vi "test Major Frame Instructions.vi"(8 "error in (no error)":errorcluster, 11 "BC Major Frame in":refnum<class "BC Major Frame.lvclass">) -> (0 "error out":errorcluster, 3 "BC Major Frame out":refnum<class "BC Major Frame.lvclass">)   [LabVIEW 2016, in "BC Major Frame.lvclass"]
uses:
  BC Major Frame.lvclass
  Data Pointers.ctl
  BC Major Frame.lvclass/BC Major Frame.ctl
  Dependencies/Registry/Registry.lvclass/Registry.ctl
  Frames & Messages/TypeDefs/BC Op Codes - Verbose.ctl
  Frames & Messages/TypeDefs/BC Condition Codes.ctl
  PPLs/FPGA Interface.lvlibp/FPGA Interface/FPGA Interface.lvclass
  BCI-1553 API.lvlib
  Dependencies/Registry/Registry.lvclass
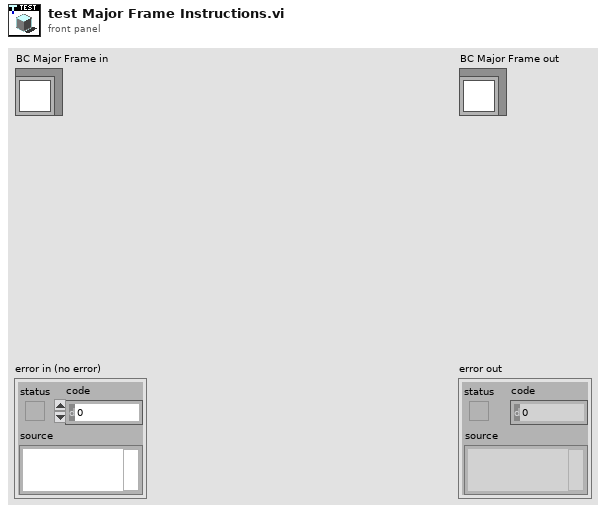
[diagram p1: front panel]
types:
  T1 = typedef "Data Pointers.ctl" = cluster{"Major Command Pointer":u16, "Major Data Pointer":u16, "Minor Command Pointer":u16, "Minor Data Pointer":u16}
  T2 = typedef "BCI-1553 API.lvlib/BC Condition Codes.ctl" = enum16{"GP0 == 1 || LT", "GP1 == 1 || NE", "GP2 == 1", "GP3 == 1", "GP4 == 1", "GP5 == 1", "GP6 == 1", "GP7 == 1", "NORESP", "FMTERR", "GOODBLOCK", "MSKSTATSET", "BADMSG", "1RETRY", "2RETRY", "ALWAYS"}
  T3 = typedef "BCI-1553 API.lvlib/BC Op Codes - Verbose.ctl" = enum16{"EXECUTE MSG", "EXECUTE MSG GO", "JUMP", "CALL SUBROUTINE", "RETURN", "INTERRUPT REQUEST", "HALT", "DELAY", "WAIT FRAME TIMER = 0", "COMPARE FRAME TIMER", "COMPARE MSG TIMER", "LOAD TIME TAG CTR", "LOAD TIME TAG CTR HI", "LOAD FRAME TIMER", "START FRAME TIMER", "PUSH TIME TAG COUNT", "PUSH TIME TAG COUNT HI", "PUSH TIME TAG COUNT BOTH", "PUSH BLOCK STATUS WORD", "PUSH CURRENT VALUE", "PUSH INDIRECT", "WAIT EXT TRIGGER", "EXECUTE AND FLIP", "EXECUTE, FLIP, GO", "WRITE VALUE TO WMI", "WRITE VALUE TO MEM", "DECREMENT RAM, SKIP", "FLAG"}
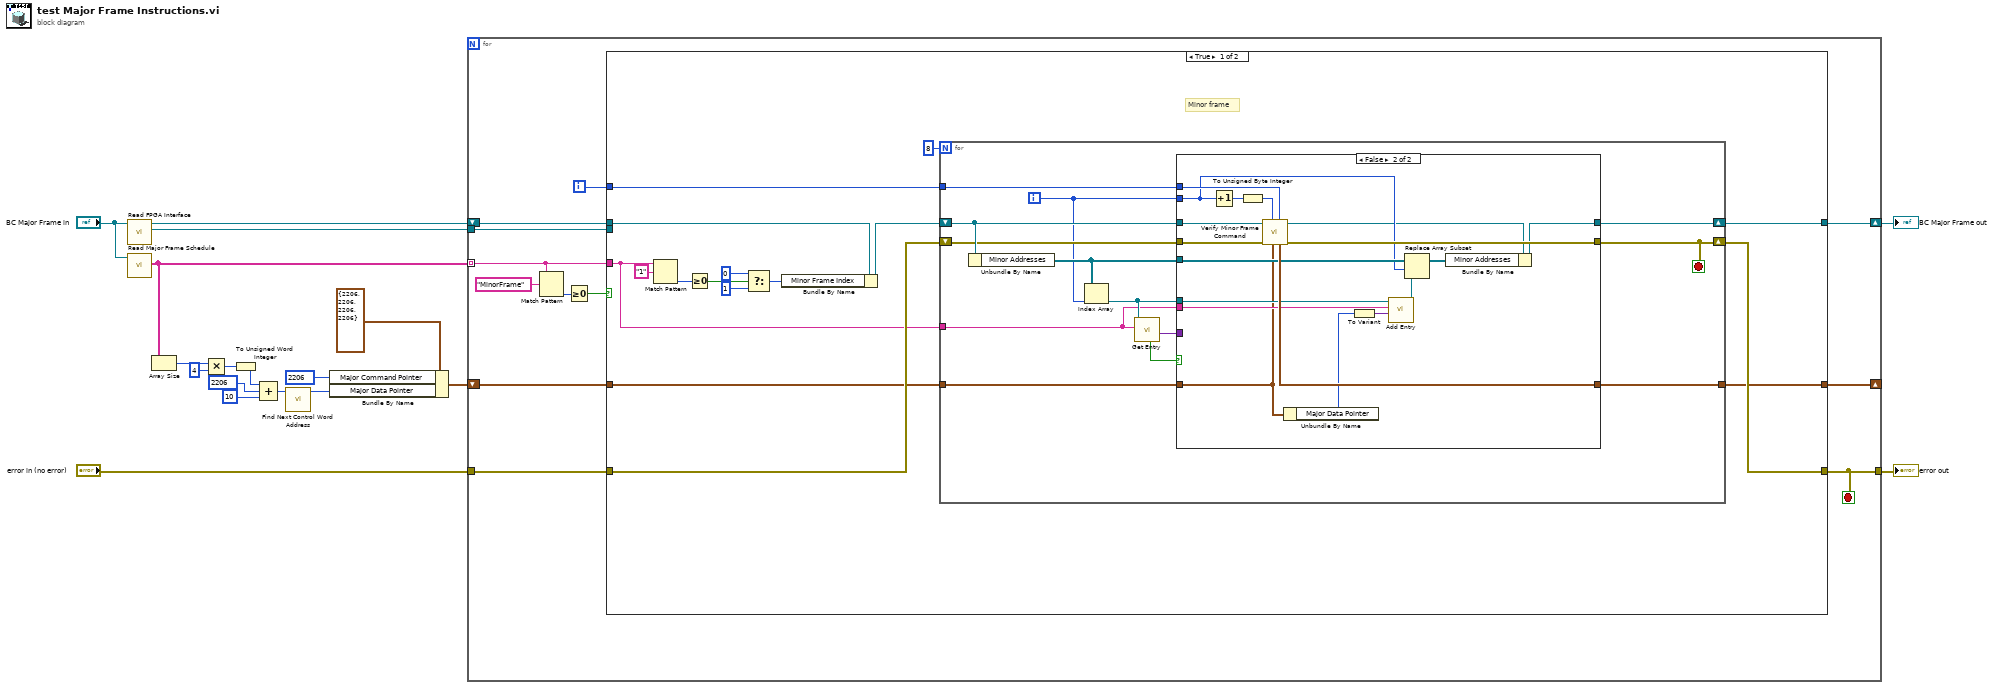
[diagram p0: block diagram]
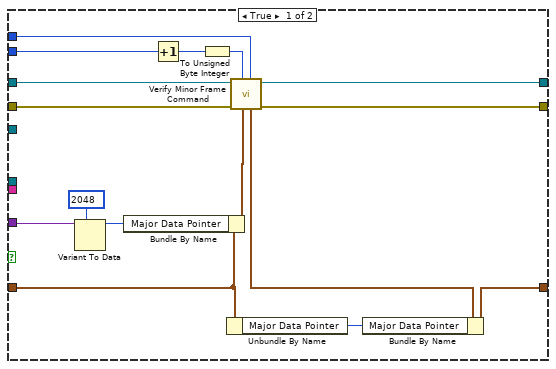
[diagram p2: hidden frame]
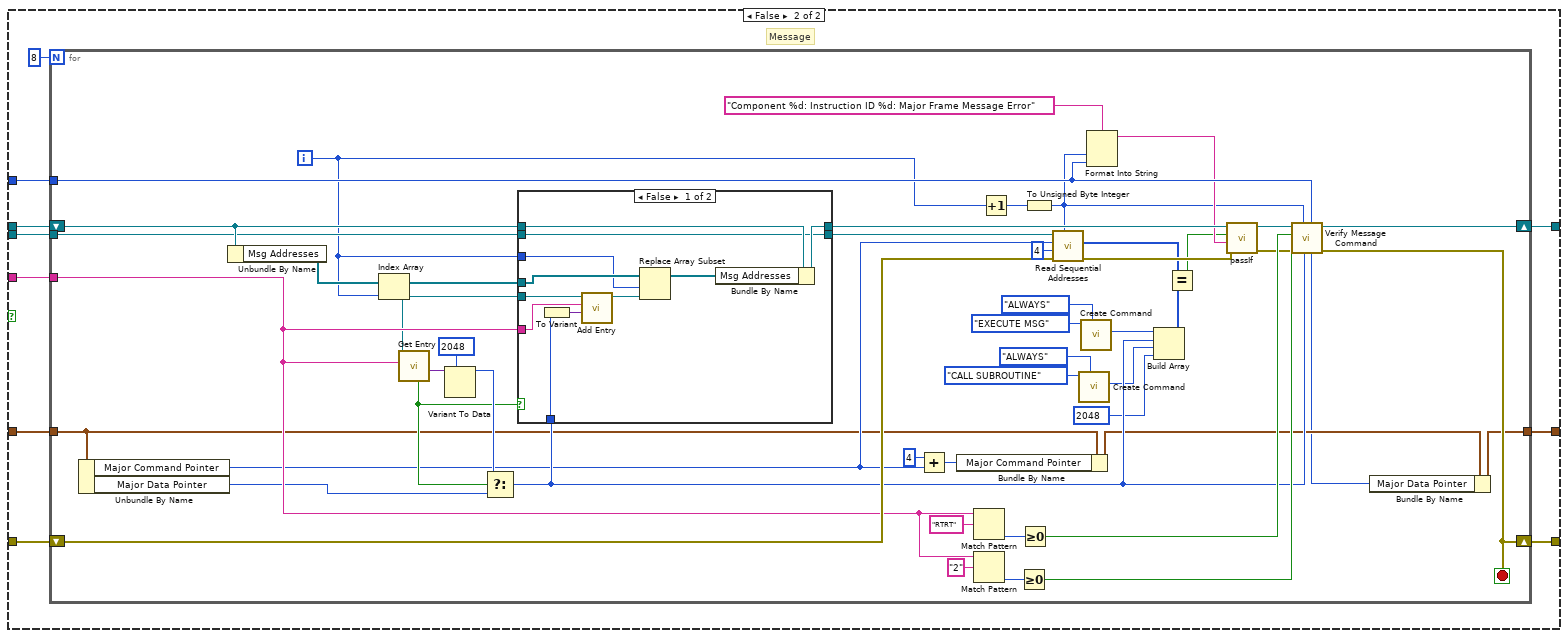
[diagram p3: hidden frame]
diagram:
  n1 = call-dynamic "Read FPGA Interface.vi"("1553 Test in"="BC Major Frame in") -> ("FPGA Interface"=w14:refnum<class "FPGA Interface.lvclass">, "1553 Test out"=w15:refnum<class "BC Major Frame.lvclass">)  [unwired: 8 in, 1 out]
  n2 = call-dynamic "Read Major Frame Schedule.vi"("1553 Test in"="BC Major Frame in") -> ("Major Frame Schedule"=w12:string[])  [unwired: 8 in, 2 out]
  n3 = Array Size(array=w12) -> (size(s)=w10:i32)
  n4 = Multiply(x=w10, y=4) -> (x*y=w8:i32)
  n5 = To Unsigned Word Integer(number=w8) -> (unsigned 16bit integer=w7:u16)
  n6 = Compound Arithmetic op=ADD(w7, u16 2206, u16 10 ("y")) -> (w5:u16)
  n7 = call "Find Next Control Word Address.vi"("Starting Address"=w5) -> ("0xHHHX Address"=w2:u16)  [unwired: 10 in]
  n8 = Bundle By Name(cluster=T1 {"Major Command Pointer"=2206, "Major Data Pointer"=2206, "Minor Command Pointer"=2206, "Minor Data Pointer"=2206}, "Major Command Pointer"=u16 2206, "Major Data Pointer"=w2) -> (w1:T1)
  n9 = for {
    shift-right: [w29] -> w18
    shift-left: w15 -> [w30]
    tunnel: "error in (no error)" -> [w28]
    tunnel: [w26] -> w16
    tunnel: w14 -> [w27]
    tunnel: w12 -> [w22] mode=indexing
    shift-right: [w19] -> _
    shift-left: w1 -> [w20]
    i -> [w21]
    stop <- w26 stop-if-true
    n10 = Match Pattern(string=w22, regular expression="MinorFrame") -> (offset past match=w24:i32)  [unwired: 1 in, 3 out]
    n11 = Greater Or Equal To 0?(x=w24) -> (x >= 0?=w23:bool)
    n12 = case shown="True" w23 {
      tunnel: w30 -> [w42 w99]
      tunnel: [w46 w103] -> w29
      tunnel: w28 -> [w44 w101]
      tunnel: [w43 w100] -> w26
      tunnel: w27 -> [_ w98]
      tunnel: w22 -> [w31 w97]
      tunnel: w21 -> [w45 w102]
      tunnel: w20 -> [w33 w95]
      tunnel: [w32 w94] -> w19
      frame True {
        # "Minor frame"
        n13 = Match Pattern(string=w31, regular expression="1") -> (offset past match=w39:i32)  [unwired: 1 in, 3 out]
        n14 = Greater Or Equal To 0?(x=w39) -> (x >= 0?=w38:bool)
        n15 = Select(t=0 ("Minor Frame Index"), s=w38, f=1 ("Minor Frame Index")) -> (s? t:f=w36:i32)
        n16 = Bundle By Name(cluster=w42, "Minor Frame Index"=w36) -> (w41:refnum<class "BC Major Frame.lvclass">)
        n17 = for {
          N: 8 -> [_]
          tunnel: w45 -> [w56]
          shift-right: [w58] -> w43
          shift-left: w44 -> [w53]
          shift-right: [w59] -> w46
          shift-left: w41 -> [w54]
          tunnel: w33 -> [w55]
          tunnel: [w57] -> w32
          tunnel: w31 -> [w47]
          i -> [w48]
          stop <- w58 stop-if-true
          n18 = Unbundle By Name(w54) -> ("Minor Addresses"=w49:refnum<class "Registry.lvclass">[])
          n19 = Index Array(array=w49, index=w48) -> (element=w50:refnum<class "Registry.lvclass">)
          n20 = call "Get Entry.vi"("Key"=w47, "Registry in"=w50) -> ("Value"=w51:variant, "Found?"=w52:bool)  [unwired: 6 in, 2 out]
          n21 = case shown="False" w52 {
            tunnel: [w75 w82] -> w59
            tunnel: [w72 w91] -> w58
            tunnel: [w61 w88] -> w57
            tunnel: w56 -> [w71 w86]
            tunnel: w55 -> [w63 w76]
            tunnel: w54 -> [w66 w89]
            tunnel: w53 -> [w70 w90]
            tunnel: w51 -> [w68 _]
            tunnel: w50 -> [_ w80]
            tunnel: w48 -> [w67 w85]
            tunnel: w49 -> [_ w87]
            tunnel: w47 -> [_ w78]
            frame True {
              n22 = Variant To Data(type=u16 2048, Variant=w68) -> (data=w65:u16)  [unwired: 1 in, 1 out]
              n23 = Bundle By Name(cluster=w63, "Major Data Pointer"=w65) -> (w64:T1)
              n24 = Increment(x=w67) -> (x+1=w73:i32)
              n25 = To Unsigned Byte Integer(number=w73) -> (unsigned 8bit integer=w74:u8)
              n26 = Unbundle By Name(w63) -> ("Major Data Pointer"=w60:u16)
              n27 = call "Verify Minor Frame Command.vi"("Instruction ID"=w71, "Pointers"=w64, "Target IC (1-8)"=w74, "error in (no error)"=w70, "BC Major Frame in"=w66) -> ("error out"=w72:errorcluster, "BC Major Frame out"=w75:refnum<class "BC Major Frame.lvclass">, "Pointers out"=w62:T1)  [unwired: 4 in]
              n28 = Bundle By Name(cluster=w62, "Major Data Pointer"=w60) -> (w61:T1)
            }
            frame False {
              n29 = Increment(x=w85) -> (x+1=w92:i32)
              n30 = To Unsigned Byte Integer(number=w92) -> (unsigned 8bit integer=w93:u8)
              n31 = call "Verify Minor Frame Command.vi"("Instruction ID"=w86, "Pointers"=w76, "Target IC (1-8)"=w93, "error in (no error)"=w90, "BC Major Frame in"=w89) -> ("error out"=w91:errorcluster, "BC Major Frame out"=w83:refnum<class "BC Major Frame.lvclass">, "Pointers out"=w88:T1)  [unwired: 4 in]
              n32 = Unbundle By Name(w76) -> ("Major Data Pointer"=w79:u16)
              n33 = To Variant(anything=w79) -> (Variant=w81:variant)
              n34 = call "Add Entry.vi"("Value"=w81, "Key"=w78, "Registry in"=w80) -> ("Registry out"=w77:refnum<class "Registry.lvclass">)  [unwired: 6 in, 2 out]
              n35 = Replace Array Subset(array=w87, new element=w77, index=w85) -> (w84:refnum<class "Registry.lvclass">[])
              n36 = Bundle By Name(cluster=w83, "Minor Addresses"=w84) -> (w82:refnum<class "BC Major Frame.lvclass">)
            }
          }
        }
      }
      frame False {
        # "Message"
        n37 = for {
          N: 8 -> [_]
          tunnel: w102 -> [w151]
          tunnel: w98 -> [w137]
          tunnel: w97 -> [w134]
          shift-right: [w111] -> w100
          shift-left: w101 -> [w150]
          shift-right: [w152] -> w103
          shift-left: w99 -> [w138]
          tunnel: w95 -> [w107]
          tunnel: [w105] -> w94
          i -> [w112]
          stop <- w111 stop-if-true
          n38 = Unbundle By Name(w107) -> ("Major Command Pointer"=w109:u16, "Major Data Pointer"=w110:u16)
          n39 = Unbundle By Name(w138) -> ("Msg Addresses"=w114:refnum<class "Registry.lvclass">[])
          n40 = Index Array(array=w114, index=w112) -> (element=w113:refnum<class "Registry.lvclass">)
          n41 = call "Get Entry.vi"("Key"=w134, "Registry in"=w113) -> ("Value"=w142:variant, "Found?"=w139:bool)  [unwired: 6 in, 2 out]
          n42 = Variant To Data(type=u16 2048, Variant=w142) -> (data=w140:u16)  [unwired: 1 in, 1 out]
          n43 = Select(t=w140, s=w139, f=w110) -> (s? t:f=w133:u16)
          n44 = case shown="False" w139 {
            tunnel: w114 -> [w155 _]
            tunnel: w134 -> [w163 _]
            tunnel: w133 -> [w162 _]
            tunnel: [w158 w165] -> w136
            tunnel: w137 -> [w158 w165]
            tunnel: [w159 w164] -> w135
            tunnel: w138 -> [w160 w164]
            tunnel: w113 -> [w157 _]
            tunnel: w112 -> [w153 _]
            frame False {
              n45 = To Variant(anything=w162) -> (Variant=w161:variant)
              n46 = call "Add Entry.vi"("Value"=w161, "Key"=w163, "Registry in"=w157) -> ("Registry out"=w156:refnum<class "Registry.lvclass">)  [unwired: 6 in, 2 out]
              n47 = Replace Array Subset(array=w155, new element=w156, index=w153) -> (w154:refnum<class "Registry.lvclass">[])
              n48 = Bundle By Name(cluster=w160, "Msg Addresses"=w154) -> (w159:refnum<class "BC Major Frame.lvclass">)
            }
            frame True {
            }
          }
          n49 = Add(x=u16 4 ("y"), y=w109) -> (x+y=w108:u16)
          n50 = Bundle By Name(cluster=w107, "Major Command Pointer"=w108) -> (w106:T1)
          n51 = Match Pattern(string=w134, regular expression="RTRT") -> (offset past match=w145:i32)  [unwired: 1 in, 3 out]
          n52 = Match Pattern(string=w134, regular expression="2") -> (offset past match=w148:i32)  [unwired: 1 in, 3 out]
          n53 = Increment(x=w112) -> (x+1=w115:i32)
          n54 = Greater Or Equal To 0?(x=w148) -> (x >= 0?=w143:bool)
          n55 = Greater Or Equal To 0?(x=w145) -> (x >= 0?=w144:bool)
          n56 = To Unsigned Byte Integer(number=w115) -> (unsigned 8bit integer=w127:u8)
          n57 = call-dynamic "Read Sequential Addresses.vi"("Target IC (1-8)"=w127, "error in (no error)"=w150, "Addresses to Read"=u16 4, "Starting Address"=w109, "FPGA Interface in"=w136) -> ("error out"=w128:errorcluster, "Data"=w118:u16[])  [unwired: 5 in]
          n58 = call "Create Command.vi"("Condition"=BC_Condition_Codes."ALWAYS", "Op Code"=BC_Op_Codes_-_Verbose."CALL SUBROUTINE") -> ("Instruction"=w121:u16)  [unwired: 8 in, 1 out]
          n59 = call "Create Command.vi"("Condition"=BC_Condition_Codes."ALWAYS", "Op Code"=BC_Op_Codes_-_Verbose."EXECUTE MSG") -> ("Instruction"=w120:u16)  [unwired: 8 in, 1 out]
          n60 = Format Into String(format string="Component %d: Instruction ID %d: Major Frame Message Error" ("message (\"\")"), w127, w151) -> (resulting string=w129:string)  [unwired: 2 in, 1 out]
          n61 = Build Array(w120, w133, w121, u16 2048) -> (w119:u16[])
          n62 = Equal?(x=w118, y=w119) -> (x = y?=w116:bool)
          n63 = call-dynamic "passIf.vi"("error in (no error)"=w128, "message (\"\")"=w129, "pass"=w116, "TestCase in"=w135) -> ("error out"=w130:errorcluster, "TestCase out"=w131:refnum<class "BC Major Frame.lvclass">)  [unwired: 6 in]
          n64 = call-dynamic "Verify Message Command.vi"("Instruction ID"=w151, "Cmd Address"=w133, "Target IC (1-8)"=w127, "error in (no error)"=w130, "Transmit?"=w143, "RT-RT?"=w144, "BC Major Frame in"=w131) -> ("error out"=w111:errorcluster, "BC Major Frame out"=w152:refnum<class "BC Major Frame.lvclass">, "Post-Data Address"=w104:u16)  [unwired: 2 in]
          n65 = Bundle By Name(cluster=w106, "Major Data Pointer"=w104) -> (w105:T1)
        }
      }
    }
  }
  "error out" <- w16
  "BC Major Frame out" <- w18
